vi "失败.vi"(1 "移动前":u16[][](array[numeric])=[[0, 0, 6, 1], [0, 0, 2, 0], [0, 0, 0, 0], [0, 0, 0, 1]]) -> (0 "失败？":bool)   [LabVIEW 2013]
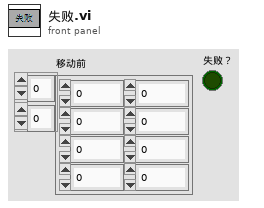
[diagram p1: front panel]
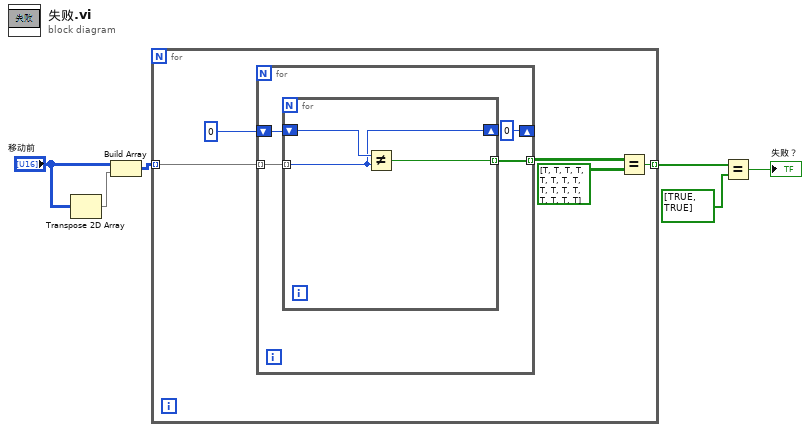
[diagram p0: block diagram]
diagram:
  n1 = Transpose 2D Array(2D array="移动前") -> (transposed array=w6:u16[][])
  n2 = Build Array("移动前", w6) -> (w5:u16[][][])
  n3 = for {
    tunnel: w5 -> [w8] mode=indexing
    tunnel: [w7] -> w4 mode=indexing
    n4 = for {
      tunnel: w8 -> [w15] mode=indexing
      shift-right: [0 ("图片")] -> _
      shift-left: 0 ("图片") -> [w14]
      tunnel: [w12] -> w10 mode=indexing
      n5 = for {
        tunnel: w15 -> [w17] mode=indexing
        shift-right: [w17] -> _
        shift-left: w14 -> [w18]
        tunnel: [w16] -> w12 mode=indexing
        n6 = Not Equal?(x=w18, y=w17) -> (x != y?=w16:bool)
      }
    }
    n7 = Equal?(x=w10, y=bool[][] [[TRUE, TRUE, TRUE, TRUE], [TRUE, TRUE, TRUE, TRUE], [TRUE, TRUE, TRUE, TRUE], [TRUE, TRUE, TRUE, TRUE]]) -> (x = y?=w7:bool)
  }
  n8 = Equal?(x=w4, y=bool[] [TRUE, TRUE]) -> (x = y?=→"失败？":bool)
